vi "EmergencyStop.vi"(0 "reference in":refnum<class "ConveyorBelt.lvclass">, 2 "Emergency":bool, 5 "error in (no error)":errorcluster) -> (14 "reference out":refnum<class "ConveyorBelt.lvclass">, 19 "error out":errorcluster)   [LabVIEW 2014, in "ConveyorBelt.lvclass"]
uses:
  ConveyorBelt.lvclass
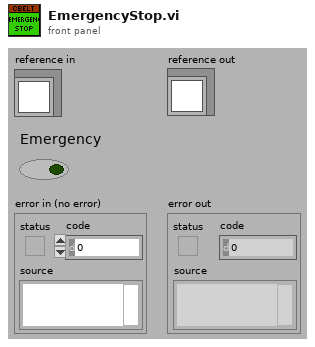
[diagram p1: front panel]
types:
  T1 = typedef "ConveyorBelt.lvclass/ObjectAttributes.ctl" = cluster{"Right":bool, "Running":bool, "ConveyorBeltRef":refnum<vi>}
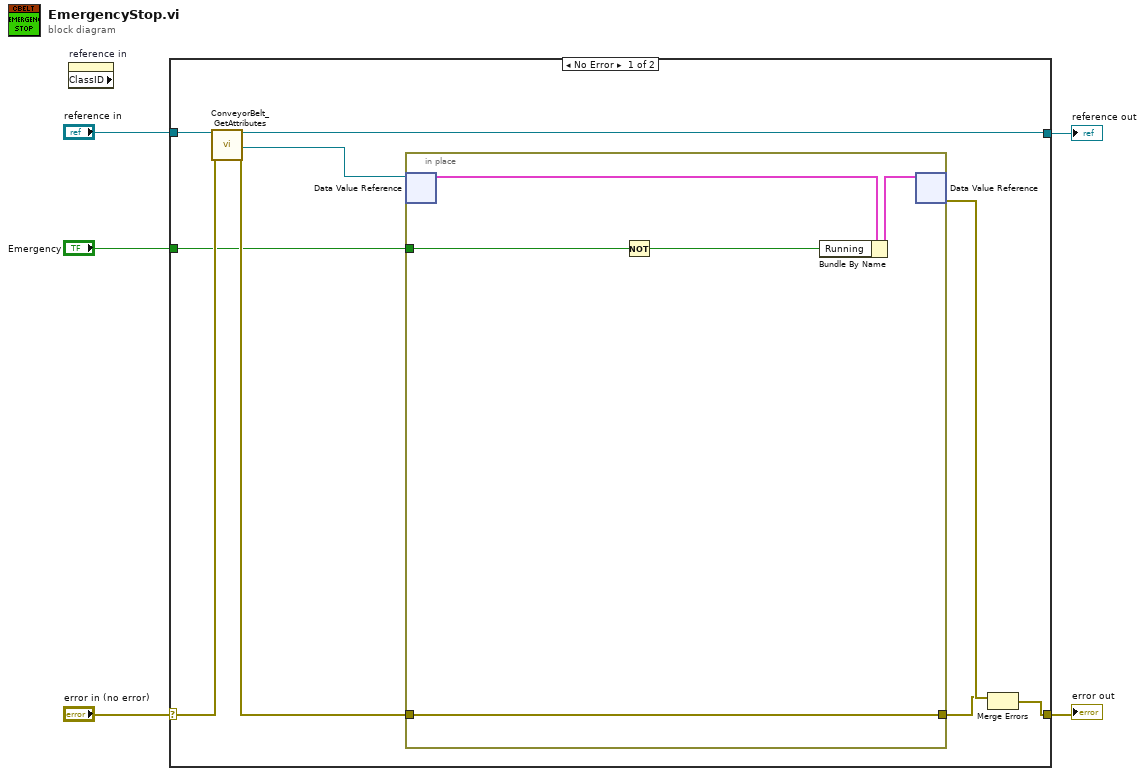
[diagram p0: block diagram]
diagram:
  n1 = property on="reference in" class="LVClassControl (strict)" props=["ClassID"]() -> ()  [unwired: 2 in, 3 out]
  n2 = case shown="No Error" "error in (no error)" {
    selector: "error in (no error)" -> [w13 w21]
    tunnel: [w10 w21] -> w4
    tunnel: [w11 w20] -> w2
    tunnel: "reference in" -> [w14 w20]
    tunnel: "Emergency" -> [w6 _]
    frame No Error {
      n3 = call "ConveyorBelt_GetAttributes.vi"("reference in"=w14, "error in (no error)"=w13) -> ("reference out"=w11:refnum<class "ConveyorBelt.lvclass">, "DataRef"=w9:refnum<data-value>, "error out"=w8:errorcluster)  [unwired: 14 in, 1 out]
      n4 = in-place {
        in-place-border: w8 -> [w17]
        in-place-border: [w17] -> w7
        in-place-border: w6 -> [w16]
        n5 = in-place-dvr #1(w9) -> (w18:T1)  [unwired: 1 out]
        n6 = Not(x=w16) -> (.not. x?=w15:bool)
        n7 = Bundle By Name(cluster=w18, "Running"=w15) -> (w19:T1)
        n8 = in-place-dvr #1(w19) -> (w12:errorcluster)  [unwired: 1 out]
      }
      n9 = Merge Errors(w12, w7) -> (w10:errorcluster)
    }
    frame Error {
    }
  }
  "error out" <- w4
  "reference out" <- w2
